vi "Import VI Snippet to Clipboard.vi"(8 "error in (no error)":errorcluster, 11 "VI Snippet (*.png)":path) -> (0 "error out":errorcluster, 1 "Copied to Clipboard?":bool)   [LabVIEW 2019]
doc: "Import a VI Snippet PNG image to the clipboard. Use the method \"VI > Diagram > Paste\" to paste the VI Snippet content. This creates a temporary VI to copy the diagram contents.\n\nCreated by: Ryan Pacini"
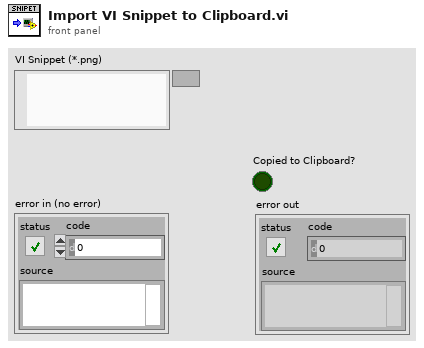
[diagram p1: front panel]
types:
  T1 = cluster{"Length":i32, "Type":string, "Data":string, "CRC":u32}[]
  T2 = cluster{"Length":i32, "Type":string, "Data":string, "CRC":u32}
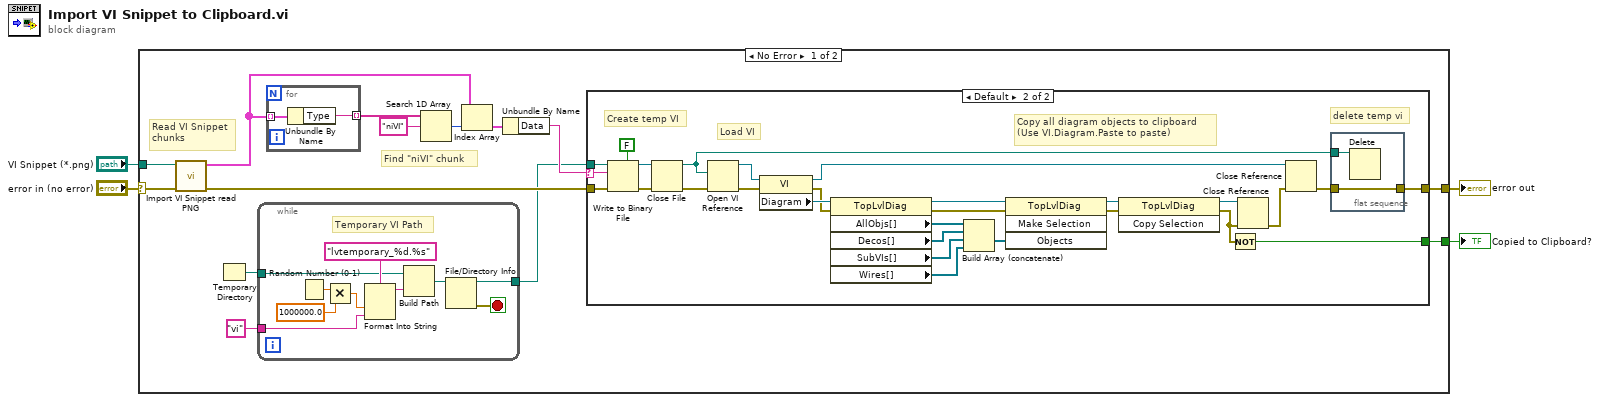
[diagram p0: block diagram]
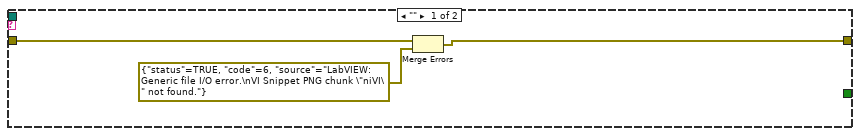
[diagram p2: hidden frame]
diagram:
  n1 = case shown="No Error" "error in (no error)" {
    selector: "error in (no error)" -> [w18 w64]
    tunnel: "VI Snippet (*.png)" -> [w17 _]
    tunnel: [w6 w64] -> w2
    tunnel: [w5 _] -> w1
    frame No Error {
      # "Read VI Snippet\nchunks"
      # "Find \"niVI\" chunk"
      n2 = call "Import VI Snippet read PNG.vi"("error in (no error)"=w18, "Path (*.png)"=w17) -> ("error out"=w10:errorcluster, "Chunks"=w13:T1)  [unwired: 8 in]
      n3 = Temporary Directory() -> (w7:path)
      n4 = while {
        tunnel: "vi" ("Temporary File Extension (tmp)") -> [w53]
        tunnel: [w54] -> w8
        tunnel: w7 -> [w52]
        stop <- w55 stop-if-true
        # "Temporary VI Path"
        n5 = Random Number (0-1)() -> (number: 0 to 1=w61:dbl)
        n6 = Multiply(x=w61, y=1000000.0) -> (x*y=w58:dbl)
        n7 = Format Into String(format string="lvtemporary_%d.%s", w58, w53) -> (resulting string=w57:string)  [unwired: 2 in, 1 out]
        n8 = Build Path(base path=w52, name or relative path=w57) -> (appended path=w56:path)
        n9 = File/Directory Info(path=w56) -> (path out=w54:path, error out=w55:errorcluster)  [unwired: 1 in, 5 out]
      }
      n10 = for {
        tunnel: w13 -> [w63] mode=indexing
        tunnel: [w62] -> w16 mode=indexing
        n11 = Unbundle By Name(w63) -> ("Type"=w62:string)
      }
      n12 = Search 1D Array(1D array=w16, element="niVI" ("Type")) -> (index of element=w14:i32)  [unwired: 1 in]
      n13 = Index Array(array=w13, index=w14) -> (element=w12:T2)
      n14 = Unbundle By Name(w12) -> ("Data"=w11:string)
      n15 = case shown="Default" w11 {
        selector: w11 -> [_ w47]
        tunnel: w10 -> [w21 w46]
        tunnel: w8 -> [_ w45]
        tunnel: [w20 w28] -> w6
        tunnel: [_ w25] -> w5
        frame "" {
          n16 = Merge Errors(w21, errorcluster {"status"=TRUE, "code"=6, "source"="LabVIEW: Generic file I/O error.\nVI Snippet PNG chunk \"niVI\" not found."} ("error in")) -> (w20:errorcluster)
        }
        frame Default {
          # "Copy all diagram objects to clipboard\n(Use VI.Diagram.Paste to paste)"
          # "delete temp vi"
          # "Load VI"
          # "Create temp VI"
          n17 = Write to Binary File(file (use dialog)=w45, data=w47, error in=w46, 5:FALSE ("prepend array or string size? (T)")) -> (refnum out=w48:refnum<file>, error out=w49:errorcluster)  [unwired: 2 in, 1 out]
          n18 = Close File(refnum=w48, error in=w49) -> (path=w29:path, error out=w43:errorcluster)
          n19 = Open VI Reference(vi path=w29, error in (no error)=w43) -> (vi reference=w24:refnum<vi>, error out=w23:errorcluster)  [unwired: 4 in]
          n20 = property class="VI"(reference=w24, error in=w23) -> (reference out=w31:refnum<vi>, error out=w41:errorcluster, "Diagram"=w42:refnum<vi>)
          n21 = property class="TopLvlDiag"(reference=w42, error in=w41) -> (reference out=w40:refnum<vi>, error out=w34:errorcluster, "AllObjs[]"=w39:refnum<vi>[], "Decos[]"=w37:refnum<vi>[], "SubVIs[]"=w36:refnum<vi>[], "Wires[]"=w35:refnum<vi>[])
          n22 = Build Array (concatenate)(w39, w37, w36, w35) -> (w38:refnum<vi>[])
          n23 = invoke class="TopLvlDiag" method="Make Selection"(reference=w40, error in=w34, "Objects"=w38) -> (reference out=w22:refnum<vi>, error out=w33:errorcluster)  [unwired: 1 in, 2 out]
          n24 = invoke class="TopLvlDiag" method="Copy Selection"(reference=w22, error in=w33) -> (reference out=w32:refnum<vi>, error out=w26:errorcluster)  [unwired: 1 in, 1 out]
          n25 = Not(x=w26) -> (.not. x?=w25:bool)
          n26 = Close Reference(reference=w32, error in (no error)=w26) -> (error out=w30:errorcluster)
          n27 = Close Reference(reference=w31, error in (no error)=w30) -> (error out=w27:errorcluster)
          n28 = flat-sequence {
            tunnel: w29 -> [w50]
            tunnel: [w51] -> w28
            tunnel: w27 -> [w51]
            frame #0 {
              n29 = Delete(path (use dialog)=w50) -> ()  [unwired: 4 in, 3 out]
            }
          }
        }
      }
    }
    frame Error {
    }
  }
  "error out" <- w2
  "Copied to Clipboard?" <- w1
